vi "Generate Report.vi"(8 "error in (no error)":errorcluster, 11 "XML Report in":refnum<class "XML Report.lvclass">) -> (0 "error out":errorcluster, 3 "XML Report out":refnum<class "XML Report.lvclass">)   [LabVIEW 2020, in "XML Report.lvclass"]
uses:
  XML Report.lvclass
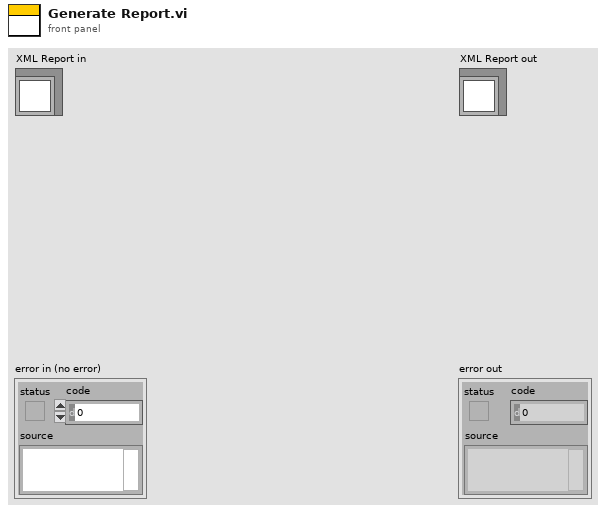
[diagram p1: front panel]
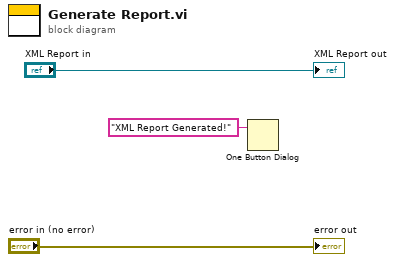
[diagram p0: block diagram]
diagram:
  n1 = One Button Dialog(message="XML Report Generated!") -> ()  [unwired: 1 in, 1 out]
  "error out" <- "error in (no error)"
  "XML Report out" <- "XML Report in"
